vi "Set Deploy Event.vi"(8 "error in (no error)":errorcluster, 10 "Deploy Event":refnum<user-event>, 11 "AppDetailPanel in":refnum<class "AppDetailPanel.lvclass">) -> (0 "error out":errorcluster, 3 "AppDetailPanel out":refnum<class "AppDetailPanel.lvclass">)   [LabVIEW 2020, in "PicoG-App.lvlib" / "AppDetailPanel.lvclass"]
uses:
  AppDetailPanel.lvclass
  Deploy Data.ctl
  ViaApp/ViaApp.lvclass
  Device/Device.lvclass
  AppDetailPanel.lvclass/AppDetailPanel.ctl
  PicoG-App.lvlib
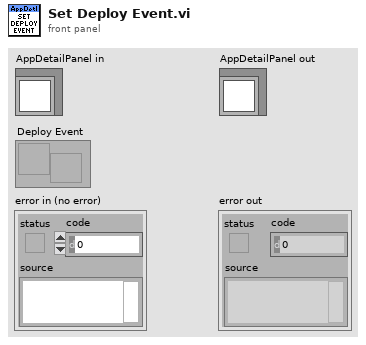
[diagram p1: front panel]
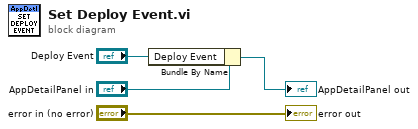
[diagram p0: block diagram]
diagram:
  n1 = Bundle By Name(cluster="AppDetailPanel in", "Deploy Event"="Deploy Event") -> (→"AppDetailPanel out":refnum<class "AppDetailPanel.lvclass">)
  "error out" <- "error in (no error)"
